vi "Get Read Write Channels.vi"(8 "error in (no error)":errorcluster, 10 "IP Address":string, 11 "Device Ref in":T2 format="%.0x") -> (0 "error out":errorcluster, 1 "Input Channel Refs":T1 {"Channel Refs" format="%.0x"}, 2 "Output Channel Refs":T1 {"Channel Refs" format="%.0x"}, 3 "Device Ref out":T2 format="%.0x")   [LabVIEW 2015, in "Shared Variable Custom Device.lvlib"]
doc: "Get the inspection's Output and Input channel references, their shared variable names, and channel types."
uses:
  Shared Variable Custom Device.lvlib
  <vilib>/NI Veristand/Custom Device API/Custom Device Item Ref.ctl
  Channel Information Control.ctl
  <vilib>/Utility/VariantDataType/Type.ctl
  Shared/Shared Variable GUID Lookup.vi
  <vilib>/NI Veristand/Custom Device Tools/Custom Device Utility Library/NI VeriStand - Search for Item by GUID.vi
  <vilib>/NI Veristand/Custom Device Tools/Custom Device Utility Library/Custom Device Utility Library.lvlib
  <vilib>/NI Veristand/Custom Device API/Custom Device API.lvlib
  <vilib>/Utility/VariantDataType/VariantType.lvlib
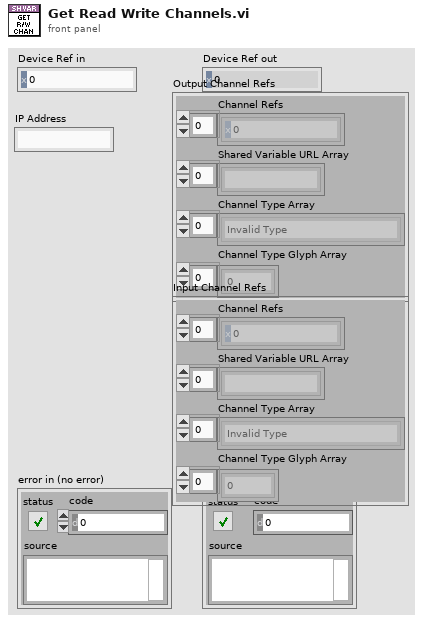
[diagram p1: front panel]
types:
  T1 = typedef "Shared Variable Custom Device.lvlib/Channel Information Control.ctl" = cluster{"Channel Refs":T2[], "Shared Variable URL Array":string[], "Channel Type Array":T3[], "Channel Type Glyph Array":i32[]}
  T2 = typedef "Custom Device API.lvlib/Custom Device Item Ref.ctl" = u64
  T3 = typedef "VariantType.lvlib/Type.ctl" = enum8{"Invalid Type", "Void", "I8", "I16", "I32", "I64", "U8", "U16", "U32", "U64", "Single Float", "Double Float", "Extended Float", "Single Complex", "Double Complex", "Extended Complex", "Enum U8", "Enum U16", "Enum U32", "Enum U64", "Single Float With Unit", "Double Float With Unit", "Extended Float With Unit", "Single Complex with Unit", "Double Complex with Unit", "Extended Complex with Unit", "Boolean", "String", "Path", "Picture", "Tag", "Array", "Cluster", "Variant", "LV Variant", "Waveform", "Timestamp", "Digital Waveform", "Digital Data", "ExpressData", "Refnum", "External Data", "VI", "Poly VI", "LabVIEW Class Instance", "Fixed Point"}
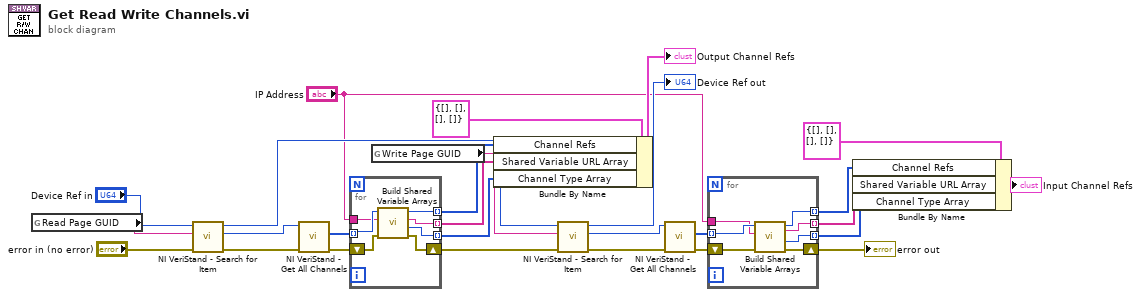
[diagram p0: block diagram]
diagram:
  n1 = global read "Shared Variable GUID Lookup.vi" "Read Page GUID"() -> (w16:string)
  n2 = call-poly <vilib>:"NI VeriStand - Search for Item.vi"("error in"="error in (no error)", "Item GUID"=w16, "Section Ref in"="Device Ref in") -> ("error out"=w23:errorcluster, "Item Ref"=w25:T2, "Section Ref out"=w11:T2)  [unwired: 5 in, 1 out]
  n3 = call <vilib>:"NI VeriStand - Get All Channels.vi"("error in"=w23, "Section Ref in"=w25) -> ("error out"=w24:errorcluster, "Channel Refs"=w22:T2[])  [unwired: 6 in, 2 out]
  n4 = for {
    tunnel: w22 -> [w33] mode=indexing
    shift-right: [w32] -> w8
    shift-left: w24 -> [w34]
    tunnel: "IP Address" -> [w31]
    tunnel: [w30] -> w20 mode=indexing
    tunnel: [w29] -> w18 mode=indexing
    tunnel: [w28] -> w17 mode=indexing
    n5 = call "Build Shared Variable Arrays.vi"("error in (no error)"=w34, "IP Address"=w31, "Channel Ref in"=w33) -> ("error out"=w32:errorcluster, "Channel Type"=w28:T3, "Shared Variable URL"=w29:string, "Channel Ref out"=w30:T2)  [unwired: 5 in]
  }
  n6 = global read "Shared Variable GUID Lookup.vi" "Write Page GUID"() -> (w7:string)
  n7 = Bundle By Name(cluster=T1 {"Channel Refs"=[], "Shared Variable URL Array"=[], "Channel Type Array"=[], "Channel Type Glyph Array"=[]} ("Input Channel Refs"), "Channel Refs"=w20, "Shared Variable URL Array"=w18, "Channel Type Array"=w17) -> (→"Output Channel Refs":T1)
  n8 = call-poly <vilib>:"NI VeriStand - Search for Item.vi"("error in"=w8, "Item GUID"=w7, "Section Ref in"=w11) -> ("error out"=w14:errorcluster, "Item Ref"=w12:T2, "Section Ref out"=→"Device Ref out":T2)  [unwired: 5 in, 1 out]
  n9 = call <vilib>:"NI VeriStand - Get All Channels.vi"("error in"=w14, "Section Ref in"=w12) -> ("error out"=w13:errorcluster, "Channel Refs"=w15:T2[])  [unwired: 6 in, 2 out]
  n10 = for {
    tunnel: w15 -> [w40] mode=indexing
    shift-right: [w39] -> w2
    shift-left: w13 -> [w41]
    tunnel: "IP Address" -> [w38]
    tunnel: [w37] -> w5 mode=indexing
    tunnel: [w36] -> w4 mode=indexing
    tunnel: [w35] -> w3 mode=indexing
    n11 = call "Build Shared Variable Arrays.vi"("error in (no error)"=w41, "IP Address"=w38, "Channel Ref in"=w40) -> ("error out"=w39:errorcluster, "Channel Type"=w35:T3, "Shared Variable URL"=w36:string, "Channel Ref out"=w37:T2)  [unwired: 5 in]
  }
  "error out" <- w2
  n12 = Bundle By Name(cluster=T1 {"Channel Refs"=[], "Shared Variable URL Array"=[], "Channel Type Array"=[], "Channel Type Glyph Array"=[]} ("Input Channel Refs"), "Channel Refs"=w5, "Shared Variable URL Array"=w4, "Channel Type Array"=w3) -> (→"Input Channel Refs":T1)
